vi "PID Gain.vi"(7 "Set? (F:Read)":bool, 8 "Error In":errorcluster, 9 "Gain (0%)":dbl, 11 "VISA resource name":refnum<visa-resource-name>) -> (0 "Error Out":errorcluster, 1 "Gain out":dbl, 3 "dup VISA resource name":refnum<visa-resource-name>)   [LabVIEW 2011, in "MGC647C.lvlib"]
doc: "Read/Set PID gain parameter."
uses:
  <instrlib>/MGC647C/MGC647C.lvlib
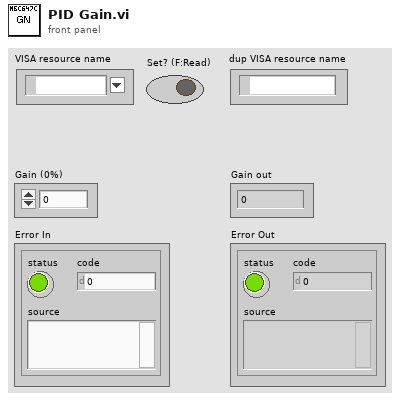
[diagram p1: front panel]
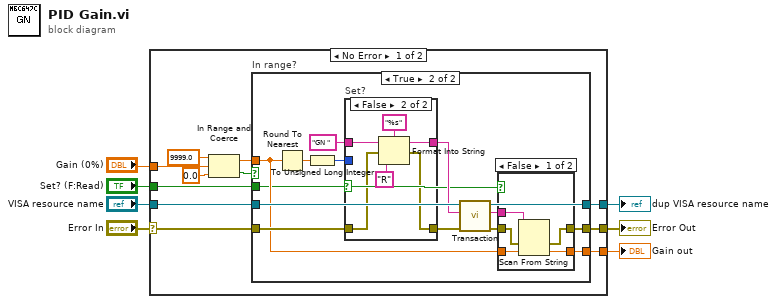
[diagram p0: block diagram]
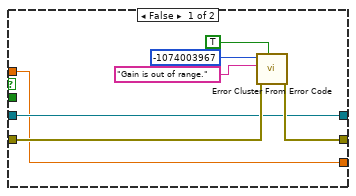
[diagram p2: hidden frame]
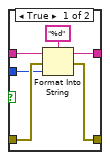
[diagram p4: hidden frame]
diagram:
  n1 = case shown="No Error" "Error In" {
    selector: "Error In" -> [w10 w60]
    tunnel: "VISA resource name" -> [w18 w59]
    tunnel: [w17 w59] -> w6
    tunnel: [w16 w60] -> w5
    tunnel: "Set? (F:Read)" -> [w15 _]
    tunnel: "Gain (0%)" -> [w14 w61]
    tunnel: [w9 w61] -> w1
    frame No Error {
      n2 = In Range and Coerce(upper limit=9999.0, x=w14, lower limit=0.0) -> (coerced(x)=w13:dbl, In Range?=w8:bool)
      n3 = case "In range?" shown="True" w8 {
        tunnel: w18 -> [w23 w39]
        tunnel: [w23 w38] -> w17
        tunnel: [w24 w33] -> w16
        tunnel: w15 -> [_ w26]
        tunnel: w13 -> [w22 w28]
        tunnel: w10 -> [w25 w37]
        tunnel: [w22 w27] -> w9
        frame False {
          n4 = call <vilib>:"Error Cluster From Error Code.vi"("show call chain? (False)"=TRUE, "error in (no error)"=w25, "error message (\"\")"="Gain is out of range." ("error message (\"\")"), "error code (0)"=-1074003967) -> ("error out"=w24:errorcluster)  [unwired: 5 in]
        }
        frame True {
          n5 = Round To Nearest(number=w28) -> (nearest integer value=w32:dbl)
          n6 = To Unsigned Long Integer(number=w32) -> (unsigned 32bit integer=w31:u32)
          n7 = case "Set?" shown="False" w26 {
            tunnel: w37 -> [w52 w58]
            tunnel: [w51 w57] -> w36
            tunnel: w31 -> [w50 _]
            tunnel: "GN " ("string (\"\")") -> [w49 w56]
            tunnel: [w48 w55] -> w29
            frame True {
              n8 = Format Into String(format string="%d", initial string=w49, error in=w52, w50) -> (resulting string=w48:string, error out=w51:errorcluster)
            }
            frame False {
              n9 = Format Into String(format string="%s", initial string=w56, error in=w58, "R") -> (resulting string=w55:string, error out=w57:errorcluster)
            }
          }
          n10 = call <instrlib>:"Transaction.vi"("Error In"=w36, "Command"=w29, "VISA resource name"=w39) -> ("Error Out"=w34:errorcluster, "Response"=w35:string, "dup VISA resource name"=w38:refnum<visa-resource-name>)  [unwired: 6 in]
          n11 = case shown="False" w26 {
            tunnel: w35 -> [w44 _]
            tunnel: w34 -> [w43 w46]
            tunnel: [w42 w46] -> w33
            tunnel: w28 -> [w41 w45]
            tunnel: [w40 w45] -> w27
            frame False {
              n12 = Scan From String(input string=w44, error in=w43, default 1=w41) -> (error out=w42:errorcluster, output 1=w40:dbl)  [unwired: 2 in, 2 out]
            }
            frame True {
            }
          }
        }
      }
    }
    frame Error {
    }
  }
  "dup VISA resource name" <- w6
  "Error Out" <- w5
  "Gain out" <- w1
